vi "RSZVB Add Ripple Limit Line Ranges Segment.vi"(4 "Type (2: Lower)":i32[](array[numeric]), 5 "Limit (none)":dbl[](array[numeric]) format="%^.3e", 6 "Stop Stimulus (none)":dbl[](array[numeric]) format="%^.3e", 7 "Start Stimulus (none)":dbl[](array[numeric]) format="%^.3e", 8 "error in (no error)":errorcluster {"code" format="%.0x"}, 9 "No of Values (1)":i32=1, 10 "Channel (Trace) (1)":i32=1, 11 "VISA session":refnum<visa-resource-name>) -> (0 "error out":errorcluster {"code" format="%.0x"}, 3 "dup VISA session":refnum<visa-resource-name>)   [LabVIEW 2011]
doc: "This VI adds and enables/disables an arbitrary number of ripple limit ranges, assigning the stimulus values and the ripple limits.\n\nNote(s):\n\nThis VI does not overwrite existing ripple limit ranges. The defined ranges are appended to the range list as new ranges. \n\n\nRemote-control command(s):\nCALCulate<Chn>:RIPPle:DATA <type>, <start_stim>, <stop_stim>, <limit>{,<type>, <start_stim>, <stop_stim>, <limit>}"
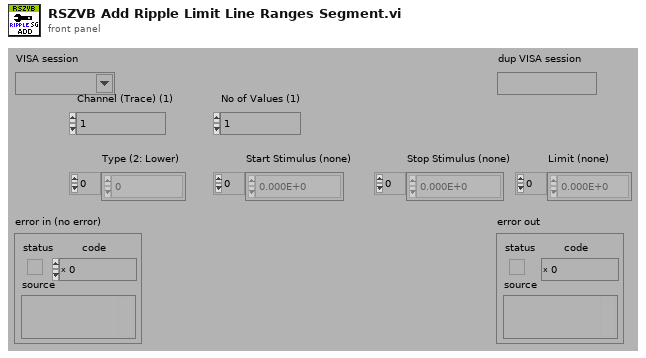
[diagram p1: front panel]
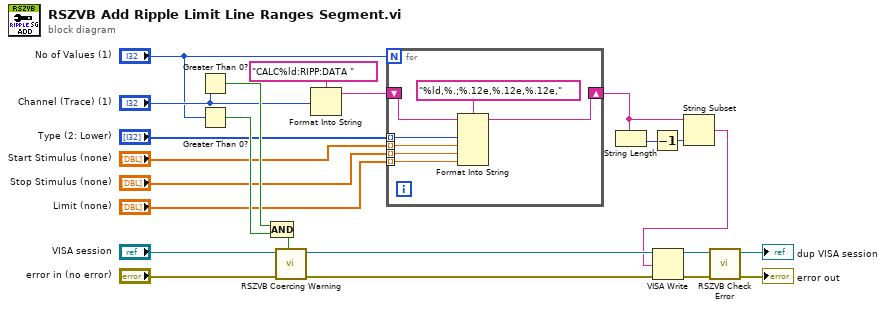
[diagram p0: block diagram]
diagram:
  n1 = Greater Than 0?(x="Channel (Trace) (1)") -> (x > 0?=w18:bool)
  n2 = Greater Than 0?(x="No of Values (1)") -> (x > 0?=w17:bool)
  n3 = Compound Arithmetic op=AND(w18, w17) -> (w19:bool)
  n4 = call "RSZVB Coercing Warning.vi"("In Range?"=w19, "error in (no error)"="error in (no error)", "VISA session"="VISA session") -> ("error out"=w22:errorcluster, "dup VISA session"=w23:refnum<visa-resource-name>)  [unwired: 7 in]
  n5 = Format Into String(format string="CALC%ld:RIPP:DATA ", "Channel (Trace) (1)") -> (resulting string=w5:string)  [unwired: 2 in, 1 out]
  n6 = for {
    N: "No of Values (1)" -> [_]
    tunnel: "Type (2: Lower)" -> [w29] mode=indexing
    tunnel: "Start Stimulus (none)" -> [w28] mode=indexing
    tunnel: "Stop Stimulus (none)" -> [w27] mode=indexing
    tunnel: "Limit (none)" -> [w26] mode=indexing
    shift-right: [w24] -> w2
    shift-left: w5 -> [w25]
    n7 = Format Into String(format string="%ld,%.;%.12e,%.12e,%.12e,", initial string=w25, w29, w28, w27, w26) -> (resulting string=w24:string)  [unwired: 1 in, 1 out]
  }
  n8 = String Length(string=w2) -> (length=w4:i32)
  n9 = Decrement(x=w4) -> (x-1=w3:i32)
  n10 = String Subset(string=w2, length (rest)=w3) -> (substring=w1:string)  [unwired: 1 in]
  n11 = VISA Write(VISA resource name=w23, write buffer=w1, error in (no error)=w22) -> (VISA resource name out=w20:refnum<visa-resource-name>, error out=w21:errorcluster)  [unwired: 1 out]
  n12 = call "RSZVB Check Error.vi"("error in (no error)"=w21, "VISA session"=w20) -> ("error out"=→"error out":errorcluster, "dup VISA session"=→"dup VISA session":refnum<visa-resource-name>)  [unwired: 8 in]
